vi "Check if configuration files exist.vi"(8 "error in (no error)":errorcluster, 11 "MeritFactorBase in":refnum<class "MeritFactor.lvclass">) -> (0 "error out":errorcluster, 2 "configuration file exists?":bool, 3 "MeritFactorBase out":refnum<class "MeritFactor.lvclass">)   [LabVIEW 2012, in "MeritFactor.lvclass"]
doc: "Checks whether all required configuration files for the component exist."
uses:
  MeritFactor.lvclass
  <vilib>/Distrio/Murmex/Murmex/Murmex.lvclass
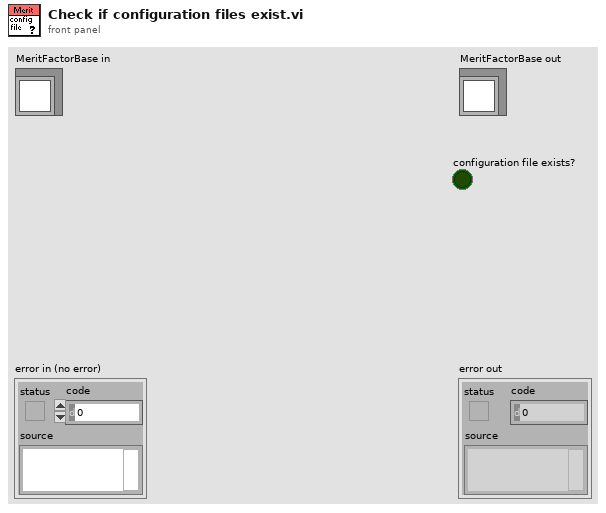
[diagram p1: front panel]
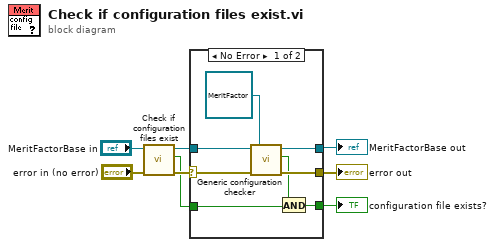
[diagram p0: block diagram]
diagram:
  n1 = call-parent "Check if configuration files exist.vi"("error in (no error)"="error in (no error)", "MurmexBase in"="MeritFactorBase in") -> ("error out"=w6:errorcluster, "configuration file exists?"=w5:bool, "MurmexBase out"=w2:refnum<class "MeritFactor.lvclass">)  [unwired: 7 in]
  n2 = case shown="No Error" w6 {
    selector: w6 -> [w14 w18]
    tunnel: w5 -> [w16 w17]
    tunnel: [w15 w17] -> w4
    tunnel: [w13 w18] -> w3
    tunnel: w2 -> [w11 w19]
    tunnel: [w10 w19] -> w1
    frame No Error {
      n3 = call <vilib>:"Generic configuration checker.vi"("error in (no error)"=w14, "inheritance level"=refnum<class "MeritFactor.lvclass"> refnum ("MeritFactor"), "Murmex in"=w11) -> ("error out"=w13:errorcluster, "configuration file exists?"=w9:bool, "Murmex out"=w10:refnum<class "MeritFactor.lvclass">)  [unwired: 6 in]
      n4 = And(x=w9, y=w16) -> (x .and. y?=w15:bool)
    }
    frame Error {
    }
  }
  "error out" <- w3
  "MeritFactorBase out" <- w1
  "configuration file exists?" <- w4
